vi "POP_Get Control Value.vi"(7 "Prop Type":T1=enum."Unkown", 8 "error in (no error)":errorcluster, 11 "Control":refnum<vi>) -> (0 "error out":errorcluster, 2 "Value":variant, 3 "dup ref":refnum<vi>)   [LabVIEW 2016]
uses:
  Ctrls/POP_Data Type.ctl
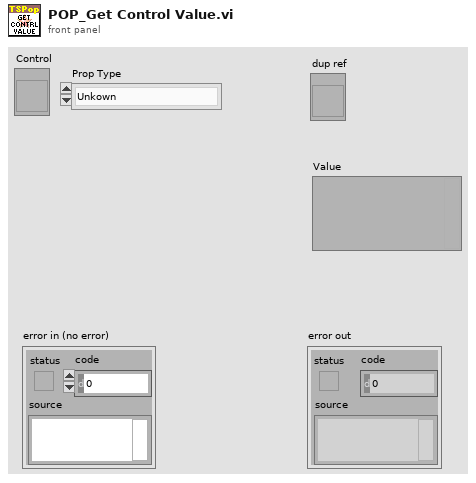
[diagram p1: front panel]
types:
  T1 = typedef "POP_Data Type.ctl" = enum16{"NO POPUP", "Unkown", "String", "Integer", "Float", "Color", "Boolean", "Ring", "Captioned String", "Captioned Integer", "Button Color", "2 Int Cluster", "4 Int Cluster", "6-Dbl Cluster", "Path", "Combox", "Time", "ShotCut String"}
  T2 = cluster{"a0":dbl, "a1":dbl, "a2":dbl, "a3":dbl, "a4":dbl, "a5":dbl}
  T3 = cluster{"left":i32, "top":i32, "right":i32, "bottom":i32}
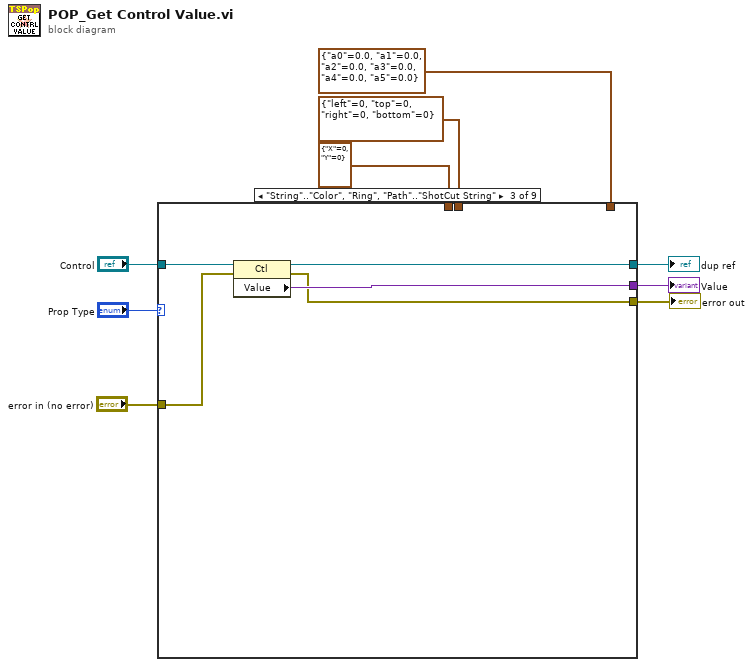
[diagram p0: block diagram]
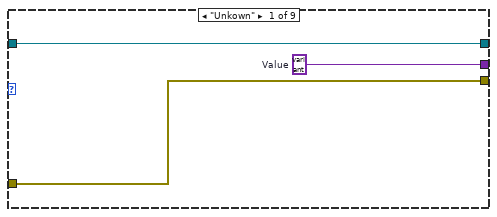
[diagram p2: hidden frame]
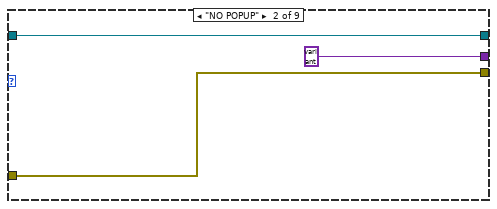
[diagram p3: hidden frame]
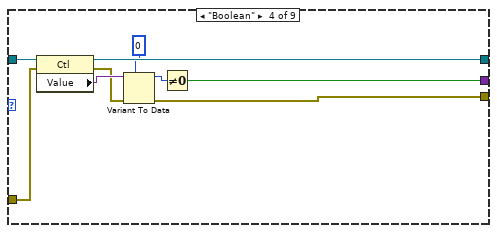
[diagram p4: hidden frame]
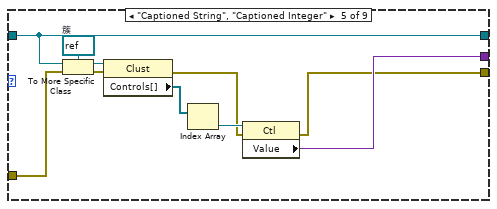
[diagram p5: hidden frame]
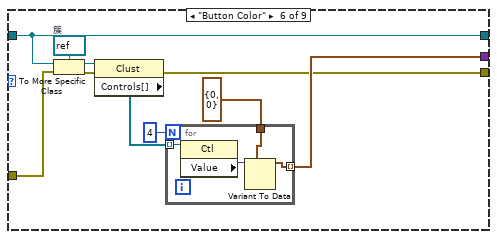
[diagram p6: hidden frame]
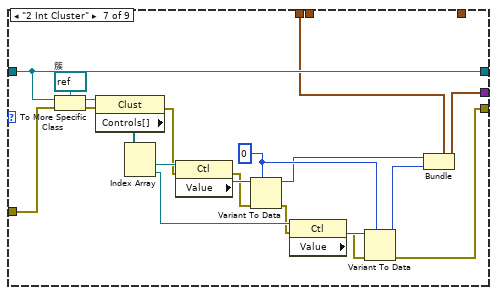
[diagram p7: hidden frame]
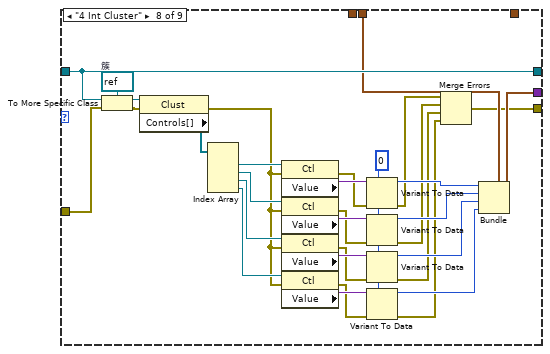
[diagram p8: hidden frame]
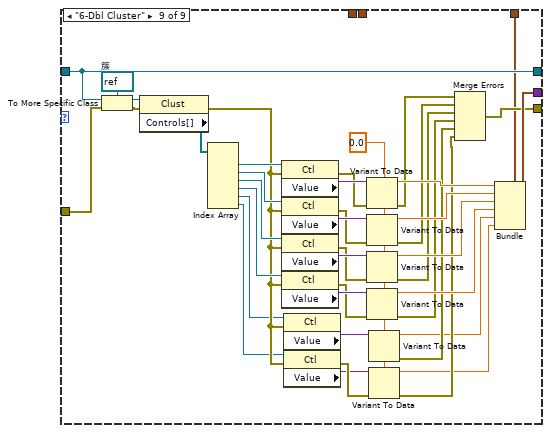
[diagram p9: hidden frame]
diagram:
  n1 = case shown="\"String\"..\"Color\", \"Ring\", \"Path\"..\"ShotCut String\"" "Prop Type" {
    tunnel: "Control" -> [w12 w15 w20 w29 w35 w44 w71 w102 w142]
    tunnel: [w12 w15 w19 w28 w35 w44 w71 w102 w142] -> w8
    tunnel: [w11 variant w18 w24 w34 w43 w61 w94 w134] -> w4
    tunnel: cluster{"X":i32, "Y":i32} {"X"=0, "Y"=0} -> [_ _ _ _ _ _ w67 _ _]
    tunnel: T3 {"left"=0, "top"=0, "right"=0, "bottom"=0} ("rect") -> [_ _ _ _ _ _ _ w93 _]
    tunnel: "error in (no error)" -> [w10 w13 w17 w23 w33 w42 w60 w85 w127]
    tunnel: [w10 w13 w16 w21 w30 w40 w54 w74 w117] -> w2
    tunnel: T2 {"a0"=0.0, "a1"=0.0, "a2"=0.0, "a3"=0.0, "a4"=0.0, "a5"=0.0} ("rect") -> [_ _ _ _ _ _ _ _ w110]
    frame "Unkown" {
      w11 = variant  # Value
    }
    frame "NO POPUP" {
    }
    frame "String".."Color", "Ring", "Path".."ShotCut String" {
      n2 = property on="Property Node" class="Ctl"(reference=w20, error in=w17) -> (reference out=w19:refnum<vi>, error out=w16:errorcluster, "Value"=w18:variant)
    }
    frame "Boolean" {
      n3 = property on="Property Node" class="Ctl"(reference=w29, error in=w23) -> (reference out=w28:refnum<vi>, error out=w22:errorcluster, "Value"=w27:variant)
      n4 = Variant To Data(error in=w22, type=0, Variant=w27) -> (data=w25:i32, error out=w21:errorcluster)
      n5 = Not Equal To 0?(x=w25) -> (x != 0?=w24:bool)
    }
    frame "Captioned String", "Captioned Integer" {
      w36 = refnum<vi> refnum  # 簇
      n6 = To More Specific Class(target class=w36, reference=w35, error in=w33) -> (specific class reference=w37:refnum<vi>, error out=w32:errorcluster)
      n7 = property class="Clust"(reference=w37, error in=w32) -> (error out=w31:errorcluster, "Controls[]"=w38:refnum<vi>[])  [unwired: 1 out]
      n8 = Index Array(array=w38) -> (element=w39:refnum<vi>)  [unwired: 1 in]
      n9 = property class="Ctl"(reference=w39, error in=w31) -> (error out=w30:errorcluster, "Value"=w34:variant)  [unwired: 1 out]
    }
    frame "Button Color" {
      w49 = refnum<vi> refnum  # 簇
      n10 = To More Specific Class(target class=w49, reference=w44, error in=w42) -> (specific class reference=w48:refnum<vi>, error out=w41:errorcluster)
      n11 = property class="Clust"(reference=w48, error in=w41) -> (error out=w40:errorcluster, "Controls[]"=w46:refnum<vi>[])  [unwired: 1 out]
      n12 = for {
        N: 4 -> [_]
        tunnel: w46 -> [w53] mode=indexing
        tunnel: cluster{u32, u32} {0, 0} -> [w51]
        tunnel: [w50] -> w43 mode=indexing
        n13 = property class="Ctl"(reference=w53) -> ("Value"=w52:variant)  [unwired: 1 in, 2 out]
        n14 = Variant To Data(type=w51, Variant=w52) -> (data=w50:cluster{u32, u32})  [unwired: 1 in, 1 out]
      }
    }
    frame "2 Int Cluster" {
      w64 = 0 ("x")
      w73 = refnum<vi> refnum  # 簇
      n15 = To More Specific Class(target class=w73, reference=w71, error in=w60) -> (specific class reference=w72:refnum<vi>, error out=w59:errorcluster)
      n16 = property class="Clust"(reference=w72, error in=w59) -> (error out=w58:errorcluster, "Controls[]"=w70:refnum<vi>[])  [unwired: 1 out]
      n17 = Index Array(array=w70) -> (element #1=w69:refnum<vi>, element #2=w68:refnum<vi>)  [unwired: 2 in]
      n18 = property class="Ctl"(reference=w69, error in=w58) -> (error out=w57:errorcluster, "Value"=w66:variant)  [unwired: 1 out]
      n19 = Variant To Data(error in=w57, type=w64, Variant=w66) -> (data=w62:i32, error out=w56:errorcluster)
      n20 = property class="Ctl"(reference=w68, error in=w56) -> (error out=w55:errorcluster, "Value"=w65:variant)  [unwired: 1 out]
      n21 = Variant To Data(error in=w55, type=w64, Variant=w65) -> (data=w63:i32, error out=w54:errorcluster)
      n22 = Bundle(cluster=w67, "X"=w62, "Y"=w63) -> (w61:cluster{"X":i32, "Y":i32})
    }
    frame "4 Int Cluster" {
      w88 = 0 ("x")
      w104 = refnum<vi> refnum  # 簇
      n23 = To More Specific Class(target class=w104, reference=w102, error in=w85) -> (specific class reference=w103:refnum<vi>, error out=w84:errorcluster)
      n24 = property class="Clust"(reference=w103, error in=w84) -> (error out=w79:errorcluster, "Controls[]"=w101:refnum<vi>[])  [unwired: 1 out]
      n25 = Index Array(array=w101) -> (element #1=w100:refnum<vi>, element #2=w99:refnum<vi>, element #3=w90:refnum<vi>, element #4=w89:refnum<vi>)  [unwired: 4 in]
      n26 = property class="Ctl"(reference=w100, error in=w79) -> (error out=w83:errorcluster, "Value"=w98:variant)  [unwired: 1 out]
      n27 = property class="Ctl"(reference=w99, error in=w79) -> (error out=w82:errorcluster, "Value"=w97:variant)  [unwired: 1 out]
      n28 = property class="Ctl"(reference=w90, error in=w79) -> (error out=w81:errorcluster, "Value"=w91:variant)  [unwired: 1 out]
      n29 = property class="Ctl"(reference=w89, error in=w79) -> (error out=w80:errorcluster, "Value"=w92:variant)  [unwired: 1 out]
      n30 = Variant To Data(error in=w83, type=w88, Variant=w98) -> (data=w95:i32, error out=w75:errorcluster)
      n31 = Variant To Data(error in=w82, type=w88, Variant=w97) -> (data=w96:i32, error out=w76:errorcluster)
      n32 = Variant To Data(error in=w81, type=w88, Variant=w91) -> (data=w87:i32, error out=w77:errorcluster)
      n33 = Variant To Data(error in=w80, type=w88, Variant=w92) -> (data=w86:i32, error out=w78:errorcluster)
      n34 = Merge Errors(w75, w76, w77, w78) -> (w74:errorcluster)
      n35 = Bundle(cluster=w93, "left"=w95, "top"=w96, "right"=w87, "bottom"=w86) -> (w94:T3)
    }
    frame "6-Dbl Cluster" {
      w105 = 0.0
      w144 = refnum<vi> refnum  # 簇
      n36 = To More Specific Class(target class=w144, reference=w142, error in=w127) -> (specific class reference=w143:refnum<vi>, error out=w126:errorcluster)
      n37 = property class="Clust"(reference=w143, error in=w126) -> (error out=w113:errorcluster, "Controls[]"=w141:refnum<vi>[])  [unwired: 1 out]
      n38 = Index Array(array=w141) -> (element #1=w140:refnum<vi>, element #2=w139:refnum<vi>, element #3=w131:refnum<vi>, element #4=w130:refnum<vi>, element #5=w107:refnum<vi>, element #6=w106:refnum<vi>)  [unwired: 6 in]
      n39 = property class="Ctl"(reference=w140, error in=w113) -> (error out=w125:errorcluster, "Value"=w138:variant)  [unwired: 1 out]
      n40 = property class="Ctl"(reference=w139, error in=w113) -> (error out=w124:errorcluster, "Value"=w137:variant)  [unwired: 1 out]
      n41 = property class="Ctl"(reference=w131, error in=w113) -> (error out=w123:errorcluster, "Value"=w132:variant)  [unwired: 1 out]
      n42 = property class="Ctl"(reference=w130, error in=w113) -> (error out=w122:errorcluster, "Value"=w133:variant)  [unwired: 1 out]
      n43 = property class="Ctl"(reference=w107, error in=w113) -> ("Value"=w115:variant)  [unwired: 2 out]
      n44 = property class="Ctl"(reference=w106, error in=w113) -> (error out=w116:errorcluster, "Value"=w114:variant)  [unwired: 1 out]
      n45 = Variant To Data(error in=w125, type=w105, Variant=w138) -> (data=w135:dbl, error out=w118:errorcluster)
      n46 = Variant To Data(error in=w124, type=w105, Variant=w137) -> (data=w136:dbl, error out=w119:errorcluster)
      n47 = Variant To Data(error in=w123, type=w105, Variant=w132) -> (data=w129:dbl, error out=w120:errorcluster)
      n48 = Variant To Data(error in=w122, type=w105, Variant=w133) -> (data=w128:dbl, error out=w121:errorcluster)
      n49 = Variant To Data(type=w105, Variant=w115) -> (data=w109:dbl, error out=w112:errorcluster)  [unwired: 1 in]
      n50 = Variant To Data(error in=w116, type=w105, Variant=w114) -> (data=w108:dbl, error out=w111:errorcluster)
      n51 = Merge Errors(w118, w119, w120, w121, w112, w111) -> (w117:errorcluster)
      n52 = Bundle(cluster=w110, "a0"=w135, "a1"=w136, "a2"=w129, "a3"=w128, "a4"=w109, "a5"=w108) -> (w134:T2)
    }
  }
  "dup ref" <- w8
  "Value" <- w4
  "error out" <- w2
